vi "Disconnect.vi"(0 "object in":refnum<class "HPS-17000-PowerModule.lvclass">, 11 "Error In":errorcluster) -> (4 "object out":refnum<class "HPS-17000-PowerModule.lvclass">, 15 "Error Out":errorcluster)   [LabVIEW 2023, in "HPS-17000-PowerModule.lvlib" / "HPS-17000-PowerModule.lvclass"]
uses:
  HPS-17000-PowerModule.lvclass
  <instrlib>/HPS-17000/Internal/Close Multi.vi
  HPS-17000-PowerModule.lvclass/HPS-17000-PowerModule.ctl
  <instrlib>/HPS-17000/HPS-17000.lvclass
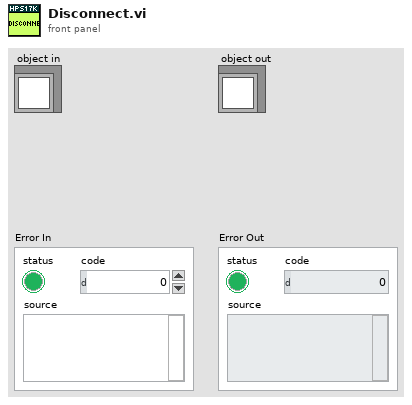
[diagram p1: front panel]
types:
  T1 = typedef "HPS-17000-PowerModule.lvlib/HPS-17000-PowerModule.lvclass/ObjectAttributes.ctl" = cluster{"JSON Config Path":path, "Configuration":T2, "GM ID":string, "HPS17000 Refs":refnum<class "HPS-17000.lvclass">[], "connected":bool, "reserved":bool, "events":T4, "nibatterycycler_grpc_Setpoint":T5, "last timestamp":i64, "mode":T6, "range":T7, "measurement array":T8[]}
  T2 = typedef "HPS-17000-PowerModule.lvlib/HPS-17000-PowerModule.lvclass/Configuration.ctl" = cluster{"TSN NIC IP Address":string, "HPS17000 IP Addresses":string[], "HPS Topology":enum16{"SINGLE", "MULTI"}, "Setpoint Stream Config":T3, "Measurement Array Size":i32}
  T3 = typedef "Cycler.lvclass/Setpoint Stream Basic Config.ctl" = cluster{"local address":string, "receiver port":u16}
  T4 = typedef "HPS-17000.lvclass/Multi-Cycler Events.ctl" = cluster{"heartbeats events":refnum<user-event>[], "faults events":refnum<user-event>[], "network sync event":refnum<user-event>[], "setpoint status event":refnum<user-event>[]}
  T5 = typedef "NI_BC_client.lvlib/nibatterycycler_grpc_Setpoint.ctl" = cluster{"voltage":sgl, "current":sgl, "min_power":sgl, "max_power":sgl, "resistance":sgl}
  T6 = typedef "HPS-17000-PowerModule.lvlib/HPS-17000-PowerModule.lvclass/Mode.ctl" = u16
  T7 = typedef "PowerModuleInterface.lvlibp/PowerModuleInterface.lvclass/Range.ctl" = cluster{"Current Max (A)":dbl, "Current Min (A)":dbl, "Voltage Max (V)":dbl, "Voltage Min (V)":dbl}
  T8 = typedef "PowerModuleInterface.lvlibp/PowerModuleInterface.lvclass/Measurements.ctl" = cluster{"measured voltage (V)":dbl, "measured current (A)":dbl, "setpoint voltage (V)":dbl, "setpoint current (A)":dbl, "timestamp":dbl}
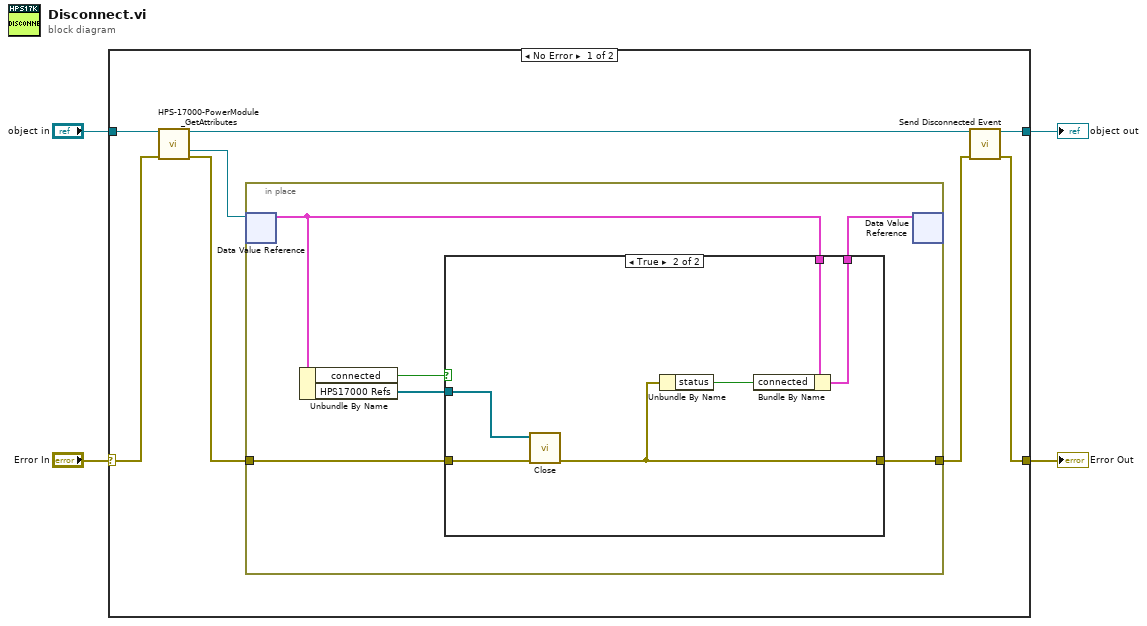
[diagram p0: block diagram]
diagram:
  n1 = case shown="No Error" "Error In" {
    selector: "Error In" -> [w11 w27]
    tunnel: "object in" -> [w12 w28]
    tunnel: [w6 w28] -> w2
    tunnel: [w5 w27] -> w3
    frame No Error {
      n2 = call "HPS-17000-PowerModule_GetAttributes.vi"("reference in"=w12, "Error In"=w11) -> ("reference out"=w7:refnum<class "HPS-17000-PowerModule.lvclass">, "DataRef"=w10:refnum<data-value>, "Error Out"=w9:errorcluster)  [unwired: 10 in, 1 out]
      n3 = in-place {
        in-place-border: w9 -> [w16]
        in-place-border: [w15] -> w8
        n4 = in-place-dvr #1(w10) -> (w17:T1)  [unwired: 1 out]
        n5 = Unbundle By Name(w17) -> ("connected"=w14:bool, "HPS17000 Refs"=w13:refnum<class "HPS-17000.lvclass">[])
        n6 = case shown="True" w14 {
          tunnel: [w20 w26] -> w18
          tunnel: w17 -> [w20 w25]
          tunnel: w16 -> [w19 w24]
          tunnel: [w19 w22] -> w15
          tunnel: w13 -> [_ w23]
          frame False {
          }
          frame True {
            n7 = call-poly <instrlib>:"Close.vi"("error in"=w24, "cycler refs in"=w23) -> ("error out"=w22:errorcluster)  [unwired: 9 in]
            n8 = Unbundle By Name(w22) -> ("status"=w21:bool)
            n9 = Bundle By Name(cluster=w25, "connected"=w21) -> (w26:T1)
          }
        }
        n10 = in-place-dvr #1(w18) -> ()  [unwired: 2 out]
      }
      n11 = call "Send Disconnected Event.vi"("reference in"=w7, "Error In"=w8) -> ("reference out"=w6:refnum<class "HPS-17000-PowerModule.lvclass">, "Error Out"=w5:errorcluster)  [unwired: 12 in]
    }
    frame Error {
    }
  }
  "Error Out" <- w3
  "object out" <- w2
